vi "AddDeviceRouting.vi"(8 "error in (no error)":errorcluster, 10 "terminal in":refnum<vi>, 11 "VI reference":refnum<vi>) -> (0 "error out":errorcluster, 3 "terminal out":refnum<vi>)   [LabVIEW 2017, in "MessageGen.lvlib"]
uses:
  <vilib>/addons/InsightCM/MessageBus/CodeGen/MessageGen.lvlib
  <vilib>/Utility/miscctls.llb/LVPointTypeDef.ctl
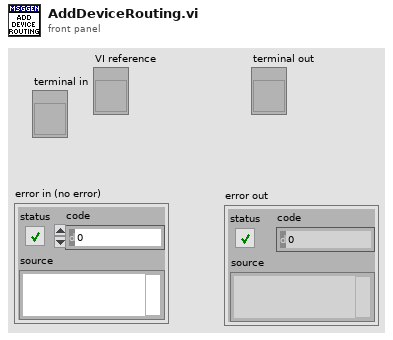
[diagram p1: front panel]
types:
  T1 = typedef "LVPointTypeDef.ctl" = cluster{"Horizontal":i16, "Vertical":i16}
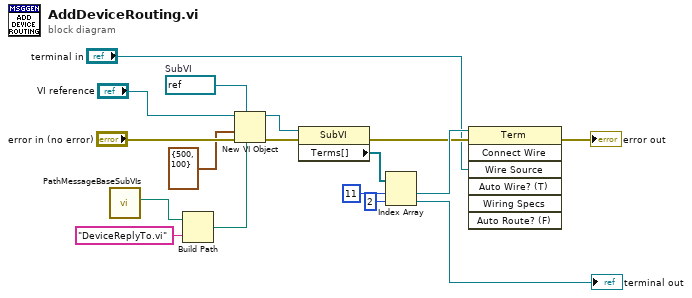
[diagram p0: block diagram]
diagram:
  w11 = refnum<vi> refnum  # SubVI
  n1 = call <vilib>:"PathMessageBaseSubVIs.vi"() -> ("Path"=w15:path)  [unwired: 11 in]
  n2 = Build Path(base path=w15, name or relative path="DeviceReplyTo.vi") -> (appended path=w13:path)
  n3 = New VI Object(vi object class=w11, owner refnum="VI reference", position/next to=T1 {"Horizontal"=500, "Vertical"=100} ("location"), 6:w13, 8:"error in (no error)") -> (object refnum=w10:refnum<vi>, 0:w9:errorcluster)  [unwired: 3 in]
  n4 = property class="SubVI"(reference=w10, error in=w9) -> (error out=w4:errorcluster, "Terms[]"=w8:refnum<vi>[])  [unwired: 1 out]
  n5 = Index Array(array=w8, index #1=11 ("index"), index #2=2 ("index")) -> (element #1=w5:refnum<vi>, element #2=→"terminal out":refnum<vi>)
  n6 = invoke class="Term" method="Connect Wire"(reference=w5, error in=w4, "Wire Source"="terminal in") -> (error out=→"error out":errorcluster)  [unwired: 4 in, 6 out]
